vi "TBM.GetCluster.vi"(8 "error in (no error)":errorcluster, 11 "Menu VI":refnum<vi>) -> (0 "error out":errorcluster, 2 "Cluster Control":refnum<vi>, 3 "Menu VI":refnum<vi>)   [LabVIEW 2013, in "ToolbarMenu.lvlib"]
uses:
  ToolbarMenu.lvlib
  <vilib>/Utility/error.llb/Error Cluster From Error Code.vi
  <vilib>/ErrorRing/Error Ring.xnode
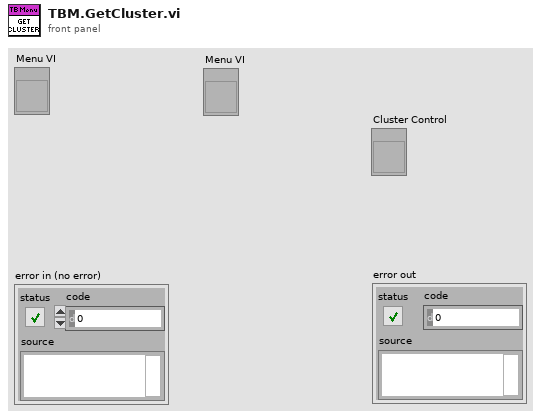
[diagram p1: front panel]
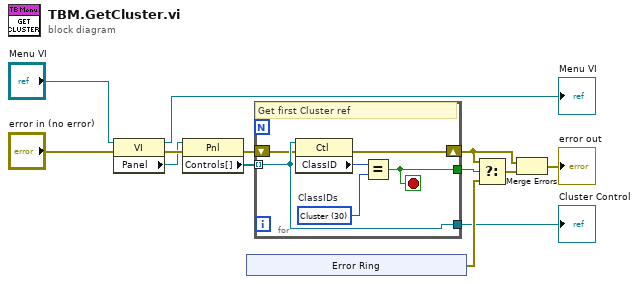
[diagram p0: block diagram]
diagram:
  n1 = property class="VI"(reference="Menu VI", error in="error in (no error)") -> (reference out=→"Menu VI":refnum<vi>, error out=w10:errorcluster, "Panel"=w9:refnum<vi>)
  n2 = property class="Pnl"(reference=w9, error in=w10) -> (error out=w13:errorcluster, "Controls[]"=w11:refnum<vi>[])  [unwired: 1 out]
  n3 = xnode "Error Ring"() -> ("error out"=w6:errorcluster)
  n4 = for {
    tunnel: w11 -> [w19] mode=indexing
    tunnel: [w19] -> w3
    shift-right: [w15] -> w8
    shift-left: w13 -> [w16]
    tunnel: [w14] -> w5
    stop <- w14 stop-if-true
    w17 = u32 30 items=["Application"=1, "VI"=2, "Generic"=3, "Decoration"=4, "Text"=5, "Control"=6, "ColorBox"=7, "Boolean"=8, "RefNum"=9, "LVVariant"=10, "Path"=11, "ListBox"=12, "Table"=13, "Array"=14, "Picture"=15, "ActiveXContainer"=16, "Numeric"=17, "Digital"=18, "NamedNumeric"=19, "ColorRamp"=20, "Slide"=21, "GraphChart"=22, "WaveformChart"=23, "WaveformGraph"=24, "IntensityChart"=25, "IntensityGraph"=26, "String"=27, "IOName"=28, "ComboBox"=29, "Cluster"=30, "Panel"=31, "Knob"=32, "NumericWithScale"=33, "Ring"=34, "Enum"=35, "GObject"=36, "Plot"=37, "Cursor"=38, "NumericText"=39, "Scale"=40, "ColorScale"=41, "GraphScale"=42, "ColorGraphScale"=43, "TypedRefNum"=44, "Generic"=45, "MulticolumnListbox"=46, "WaveformData"=47, "DSCTag"=48, "DAQChannelName"=49, "VISAResourceName"=50, "IVILogicalName"=51, "SlideScale"=52, "PageSelector"=53, "Page"=54, "TabControl"=55, "ConnectorPane"=56, "DAQmxName"=57, "VIRefNum"=58, "LVObjectRefNum"=59, "AbsTime"=60, "DigitalTable"=61, "SubsystemVI"=62, "Generic"=63, "Generic"=64, "SubPanel"=65, "TreeControl"=66, "GenClassTagRef"=67, "GenClassRef"=68, "RotaryColorScale"=69, "PlugInControl"=70, "PlugInDDODummyContainer"=71, "RadioButtonsControl"=72, "Project"=73, "ProjectItem"=74, "Pane"=75, "Splitter"=76, "BuildSpecification"=77, "Pixmap"=78, "FacadeVI"=79, "Library"=80, "Variable"=81, "TagSet"=82, "XYGraph"=83, "SceneWindow"=84, "LVClassLibrary"=85, "Generic"=86, "MethodVI"=87, "XControlLibrary"=88, "XNodeLibrary"=89, "Scrollbar"=90, "LVTarget"=91, "MixedSignalGraph"=92, "Provider"=93, "CopyOperation"=94, "TargetItem"=95, "ProjectItemType"=96, "CopyItem"=97, "CopyConflict"=98, "CopyExpert"=99, "SceneGraphDisplay"=100, "PolymorphicVI"=101, "LabVIEWClassControl"=102, "XInterfaceLibrary"=103, "SceneNode"=104, "SceneObject"=105, "SceneLight"=106, "Generic"=107, "Generic"=108, "Generic"=109, "SceneClipPlane"=110, "SceneTexture"=111, "SceneGeometry"=112, "SceneBox"=113, "SceneCone"=114, "SceneCylinder"=115, "SceneHeightField"=116, "SceneSphere"=117, "SceneMesh"=118, "XPropertyFolder"=119, "PropertyFolder"=120, "DigitalGraph"=121, "GenClassTagFlatRef"=122, "Scene"=123, "Generic"=124, "LibraryData"=125, "StatechartLibrary"=126, "MixedCheckbox"=127, "SceneDrawable"=128, "SceneText"=129, "MultiSegmentPipe"=130, "Bus"=131, "StubDDO"=132, "ProjectFilesViewItem"=133, "LVClassPropDefFolder"=134, "DataValRefNum"=135]  # ClassIDs
    # "Get first Cluster ref"
    n5 = property class="Ctl"(reference=w19, error in=w16) -> (error out=w15:errorcluster, "ClassID"=w18:u32)  [unwired: 1 out]
    n6 = Equal?(x=w18, y=w17) -> (x = y?=w14:bool)
  }
  "Cluster Control" <- w3
  n7 = Select(t=w8, s=w5, f=w6) -> (s? t:f=w7:errorcluster)
  n8 = Merge Errors(w8, w7) -> (→"error out":errorcluster)
